vi "Main.vi"() -> ()   [LabVIEW 2019]
uses:
  WorkSpace/LabVIEW/Simon - ActiveX - Version - 0.5/Control/Display.ctl
  ctl/InfoOfPlayer.ctl
panel:
  in  "结束游戏":bool
  in  "选项卡控件":enum32{"启动界面", "单机游戏界面", "多人游戏界面", "排行榜"}(tab)
  in  "选择游戏难度":u16(ring)=1000 items=["入门"=1000, "进阶"=850, "偏难"=700]
  in  "玩家昵称":string="Player"
  in  "游戏类型":enum32{"人机模式", "玩家对战"}(radio)
  in  "启动游戏":bool
  out "存档地址":path
  in  "加载存档":bool
  in  "游戏存档":bool
  out "公告":string
  in  "人机玩家信息":T1
  in  "人机游戏显示界面":T2
  in  "返回启动界面":bool
  out "排行榜路径":path
  in  "排行榜":T1[](array[typedef])
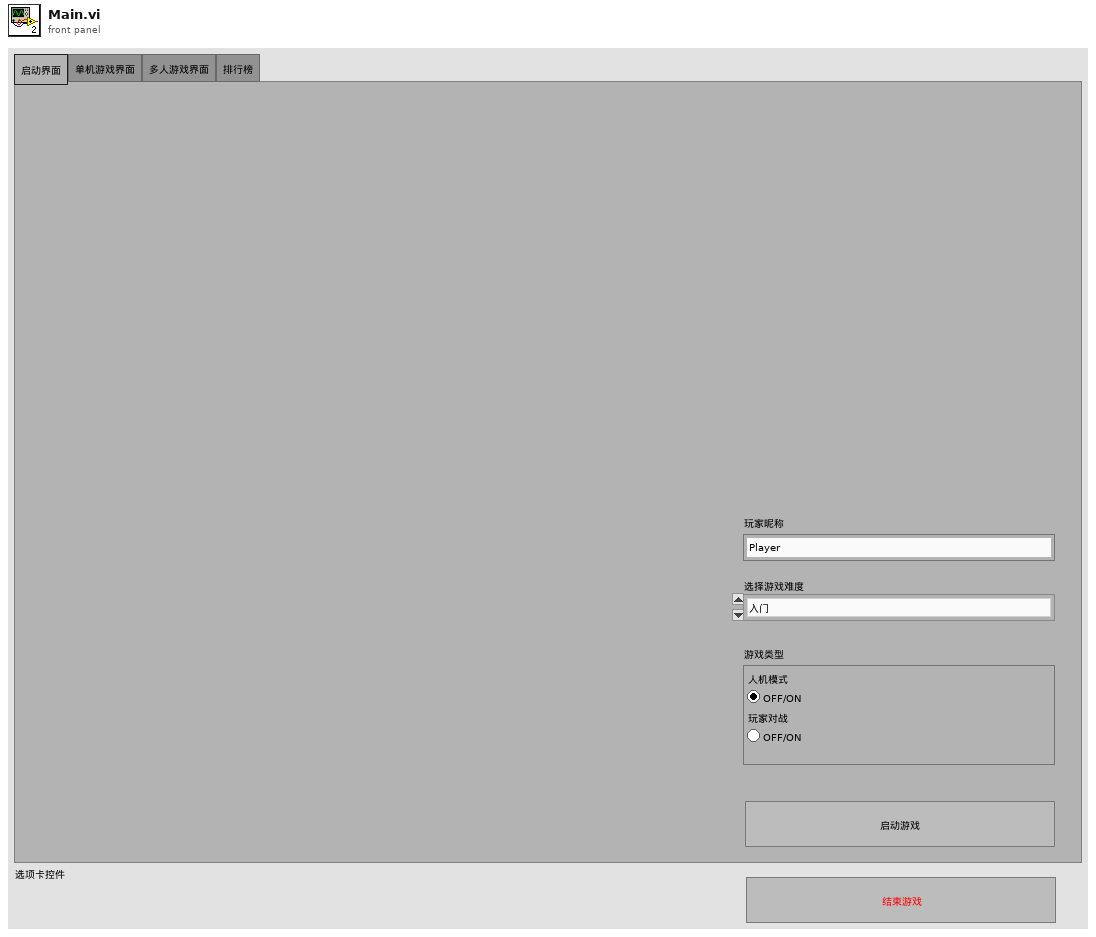
[diagram p1: front panel]
types:
  T1 = typedef "InfoOfPlayer.ctl" = cluster{"得分":i32, "英雄":string}
  T2 = typedef "Display.ctl" = cluster{"左上":bool, "右上":bool, "左下":bool, "右下":bool}
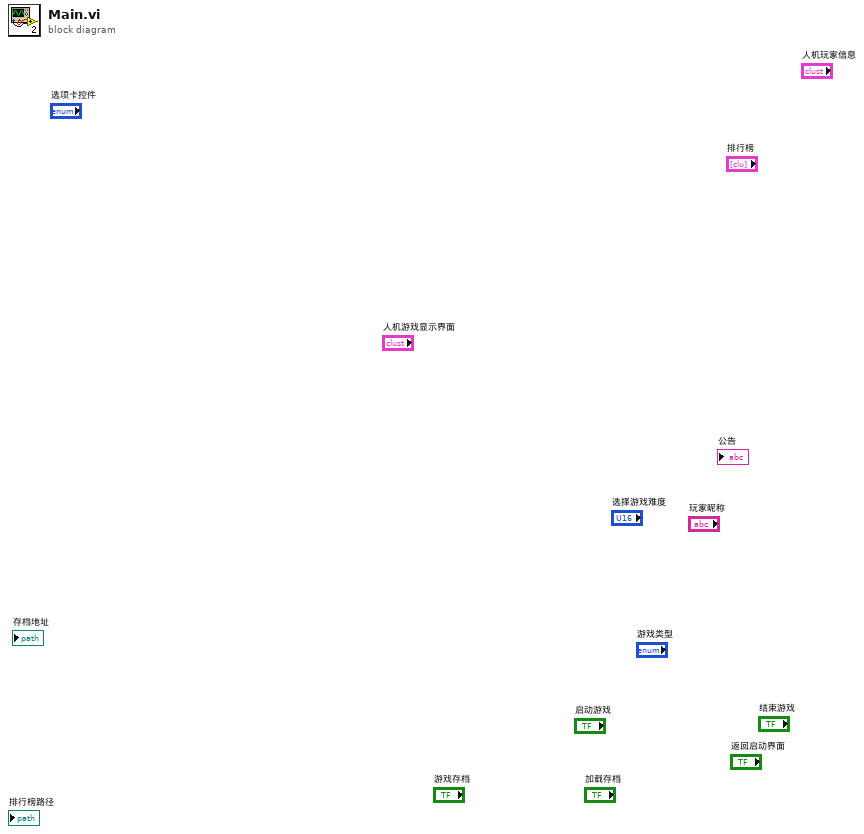
[diagram p0: block diagram]
diagram:
